vi "picoquant_read_buffer.vi"(8 "error in (no error)":errorcluster, 11 "hydraharp in":refnum<class "hydraharp.lvclass">) -> (0 "error out":errorcluster, 2 "new_data":u32[](array[numeric]), 3 "hydraharp out":refnum<class "hydraharp.lvclass">)   [LabVIEW 2015, in "hydraharp.lvclass"]
uses:
  hydraharp.lvclass
  hydraharp.lvclass/hydraharp.ctl
  hhlib.dll
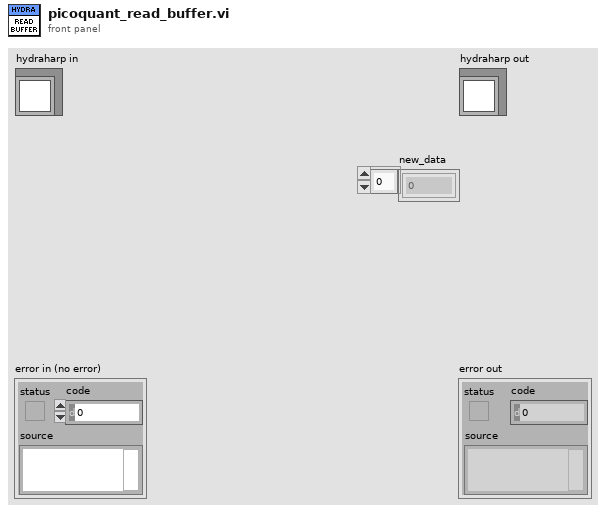
[diagram p1: front panel]
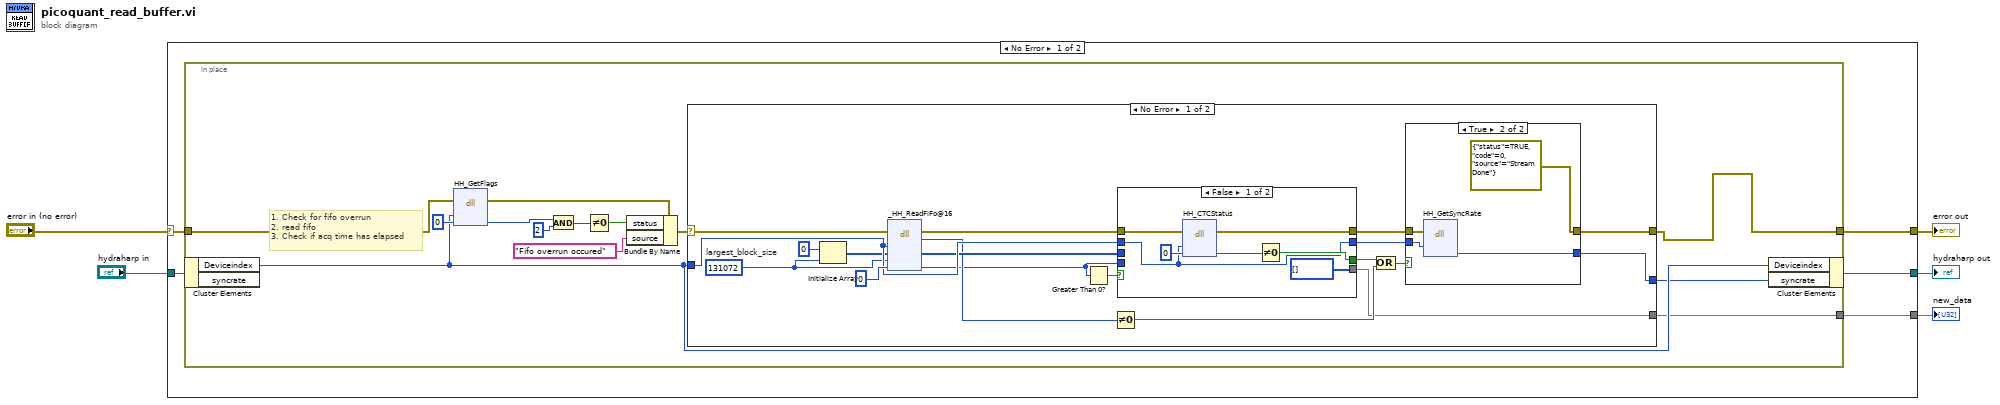
[diagram p0: block diagram]
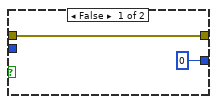
[diagram p2: hidden frame]
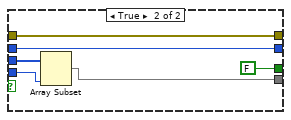
[diagram p3: hidden frame]
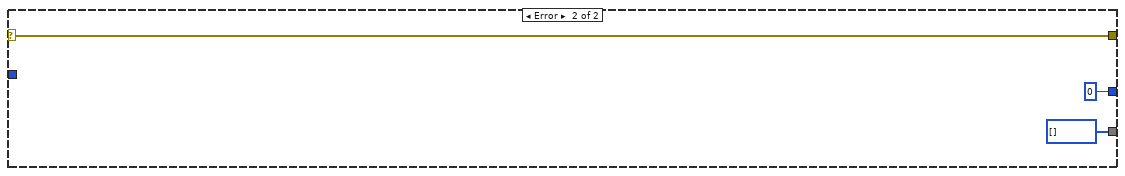
[diagram p4: hidden frame]
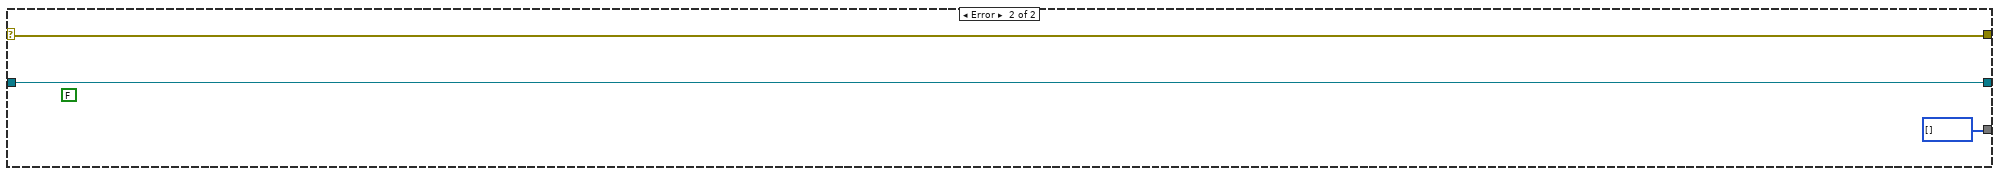
[diagram p5: hidden frame]
diagram:
  n1 = case shown="No Error" "error in (no error)" {
    selector: "error in (no error)" -> [w9 w67]
    tunnel: [w8 w67] -> w2
    tunnel: [w7 w66] -> w3
    tunnel: "hydraharp in" -> [w10 w66]
    tunnel: [w6 u32[] []] -> w1
    frame No Error {
      n2 = in-place {
        in-place-border: w9 -> [w23]
        in-place-border: [w11] -> w8
        in-place-border: [w12] -> w6
        # "1. Check for fifo overrun\n2. read fifo\n3. Check if acq time has elapsed"
        n3 = in-place-cluster #1(w10) -> ("Deviceindex"=w19:i32)  [unwired: 1 out]
        n4 = dll-call lib="hhlib.dll" fn="HH_GetFlags"(error in=w23, "devidx"=w19, "flags"=0) -> (error out=w18:errorcluster, "flags"=w21:i32)  [unwired: 4 in, 1 out]
        n5 = And(x=w21, y=2) -> (x .and. y?=w15:i32)
        n6 = Not Equal To 0?(x=w15) -> (x != 0?=w14:bool)
        n7 = Bundle By Name(cluster=w18, "status"=w14, "source"="Fifo overrun occured") -> (w16:errorcluster)
        n8 = case shown="No Error" w16 {
          selector: w16 -> [w34 w64]
          tunnel: w19 -> [w39 _]
          tunnel: [w35 w64] -> w11
          tunnel: [w25 0 ("syncrate")] -> w13
          tunnel: [w24 u32[] []] -> w12
          frame No Error {
            w28 = 131072  # largest_block_size
            n9 = Initialize Array(u32 0 ("element"), w28) -> (w27:u32[])
            n10 = dll-call lib="hhlib.dll" fn="_HH_ReadFiFo@16" label="HH_ReadFiFo"(error in=w34, "devidx"=w39, "buffer"=w27, "blocksize"=w28, "nactual"=0) -> (error out=w40:errorcluster, "return type"=w33:i32, "buffer"=w37:u32[], "nactual"=w30:i32)  [unwired: 4 in, 1 out]
            n11 = Greater Than 0?(x=w30) -> (x > 0?=w41:bool)
            n12 = Not Equal To 0?(x=w33) -> (x != 0?=w32:bool)
            n13 = case shown="False" w41 {
              tunnel: w40 -> [w55 w56]
              tunnel: [w54 w56] -> w31
              tunnel: w39 -> [w50 w58]
              tunnel: [w52 FALSE] -> w38
              tunnel: w37 -> [_ w60]
              tunnel: w30 -> [_ w59]
              tunnel: [w50 w58] -> w26
              tunnel: [u32[] [] w57] -> w24
              frame False {
                n14 = dll-call lib="hhlib.dll" fn="HH_CTCStatus"(error in=w55, "devidx"=w50, "status"=0) -> (error out=w54:errorcluster, "status"=w51:i32)  [unwired: 4 in, 1 out]
                n15 = Not Equal To 0?(x=w51) -> (x != 0?=w52:bool)
              }
              frame True {
                n16 = Array Subset(array=w60, length=w59) -> (w57:u32[])  [unwired: 1 in]
              }
            }
            n17 = Or(x=w38, y=w32) -> (x .or. y?=w36:bool)
            n18 = case shown="True" w36 {
              tunnel: w31 -> [w44 w48]
              tunnel: [w44 errorcluster {"status"=TRUE, "code"=0, "source"="Stream Done"} ("error out")] -> w35
              tunnel: w26 -> [_ w47]
              tunnel: [0 ("syncrate") w46] -> w25
              frame False {
              }
              frame True {
                n19 = dll-call lib="hhlib.dll" fn="HH_GetSyncRate"(error in=w48, "devidx"=w47) -> ("syncrate"=w46:i32)  [unwired: 5 in, 2 out]
              }
            }
          }
          frame Error {
          }
        }
        n20 = in-place-cluster #1("Deviceindex"=w19, "syncrate"=w13) -> (w7:refnum<class "hydraharp.lvclass">)
      }
    }
    frame Error {
      (unwired) FALSE
    }
  }
  "error out" <- w2
  "hydraharp out" <- w3
  "new_data" <- w1
